vi "ATS_SetTriggerTimeOut.vi"(9 "TimeX (1000)":u32=1000, 10 "Timeout (-1s)":dbl=-1.0 format="%.2f", 11 "DeviceIn":i32) -> (0 "Return Code":u32, 2 "Timeout_Set":dbl format="%.2f", 3 "DeviceOut":i32)   [LabVIEW 2015]
doc: "_____AlazarTech, Scope_____\n\nSpecify a timeout for a trigger event. If no trigger occurs in the specified amount of time, the board automatically forces a trigger.\nIn Master/Slave mode all board are set to the same value.\n\nIf Timeout input is < 0, a Timeout = Clock x Length x TimeX(100) will be used.\n\nMinimum value is 10e-6s.\nMaximum 3600s (1hour)."
uses:
  ATS_ctl/ATS_Global_Ctrl.ctl
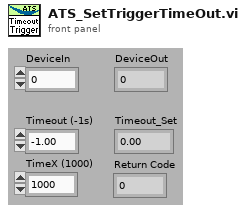
[diagram p1: front panel]
types:
  T1 = typedef "ATS_Global_Ctrl.ctl" = enum16{"Init_Device", "Clear_ALL", "Set", "Get"}
  T2 = typedef "ATS_Sys_Info.ctl" = cluster{"MS_Mode":bool, "MBoard":i32, "#Board":i32}
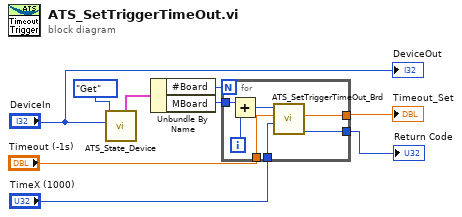
[diagram p0: block diagram]
diagram:
  n1 = call "ATS_State_Device.vi"("DeviceIn"="DeviceIn", "ATS_GBL_Ctrl"=ATS_Global_Ctrl."Get") -> ("Sys_Out"=w8:T2)  [unwired: 4 in, 5 out]
  n2 = Unbundle By Name(w8) -> ("#Board"=w7:i32, "MBoard"=w6:i32)
  n3 = for {
    N: w7 -> [_]
    tunnel: w6 -> [w15]
    tunnel: "Timeout (-1s)" -> [w13]
    tunnel: "TimeX (1000)" -> [w12]
    tunnel: [w11] -> w3
    tunnel: [w10] -> w2
    i -> [w16]
    n4 = Add(x=w15, y=w16) -> (x+y=w14:i32)
    n5 = call "ATS_SetTriggerTimeOut_Brd.vi"("TimeX (1000)"=w12, "Timeout (-1s)"=w13, "DeviceIn"=w14) -> ("Return Code"=w11:u32, "Timeout_Set"=w10:dbl)  [unwired: 6 in, 1 out]
  }
  "Return Code" <- w3
  "Timeout_Set" <- w2
  "DeviceOut" <- "DeviceIn"
